vi "PWA_Setup_Panel.vi"(0 "Show Panel?":bool, 1 "Check Calib file?":bool, 2 "OK":T1, 3 "Incoming Setup String":string) -> (7 "Outgoing Setup String":string)   [LabVIEW 2013]
uses:
  Controls/ok_button.ctl
  File/Setup_Filetype.ctl
  Controls/Post_Process.ctl
  Controls/App_Global.ctl
  Controls/Inst_type.ctl
  Globals/Meas_global.vi
  PWAtasksGLOBAL.vi
panel:
  in  "Probe Rotated Thro' 180":bool
  in  "Software + buffering delay per pulse (s)":dbl=9.7e-06
  in  "Symbol":string
  in  "Pulse length \nx2 micro sec":i16=1 min=1 max=12
  in  "Clock Rate":bool
  in  "Gain":i16=1 min=1 max=12
  in  "Wire Current mA":i16(knob)=1 min=1 max=3 step=1 scale=1.0..3.0
  in  "Trigger -ve":dbl(knob)=1.0 min=0.0 max=5.0 scale=0.0..5.0 scale format="%#.2f"
  in  "Trigger +ve":dbl(knob)=1.0 min=0.0 max=5.0 scale=0.0..5.0 scale format="%#.2f"
  out "Calib Path from file":path
  in  "Use Latest":bool=TRUE
  in  "PWA Calib. File Path":path=path "/G5_1_HD/Users/paulhayden/Desktop/Labview test/PWA_Calib.xls"
  in  "Minimum TOF (mu.s)":i16=225
  in  "PWA Freq. (Hz)":dbl=30.0 min=0.0 max=50.0
  # "PELA Flow Instruments Ltd."
  # "TRIGGER LEVELS\n(volts)"
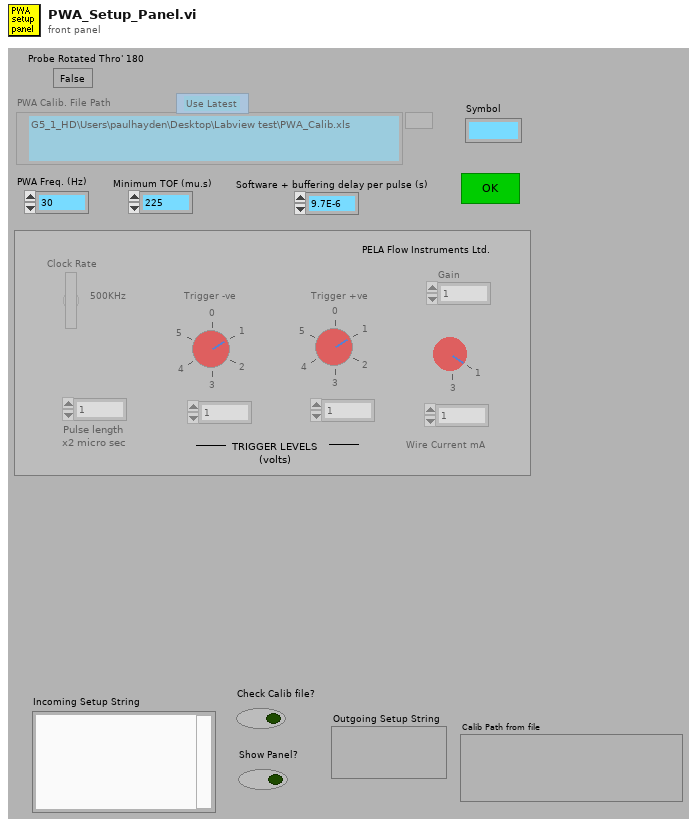
[diagram p1: front panel]
types:
  T1 = typedef "ok_button.ctl" = bool
  T2 = typedef "Setup_Filetype.ctl" = enum16{"Measurement Setups", "Calibration Setups", "General", "Results File Plotter Setups", "Speed Calib Tweaks"}
  T3 = typedef "Post_Process.ctl" = enum16{"Take New Data", "Post Process Raw Data File"}
  T4 = typedef "App_Global.ctl" = enum16{"Read Global", "Write to Global", "Initialise Array"}
  T5 = typedef "Inst_type.ctl" = enum16{"Propeller anemometer", "Raw voltage", "Pressure Transducer", "Pitot-static tube", "Preston tube", "Hot wire", "Cross wire 1", "Cross wire 2", "Generic Linear", "Generic Polynomial", "Generic BackPoly", "Fast FID", "Thermocouple", "Cold wire", "Pulsed Wire", "LDA Vel", "LDA Tran time", "LDA Arr time"}
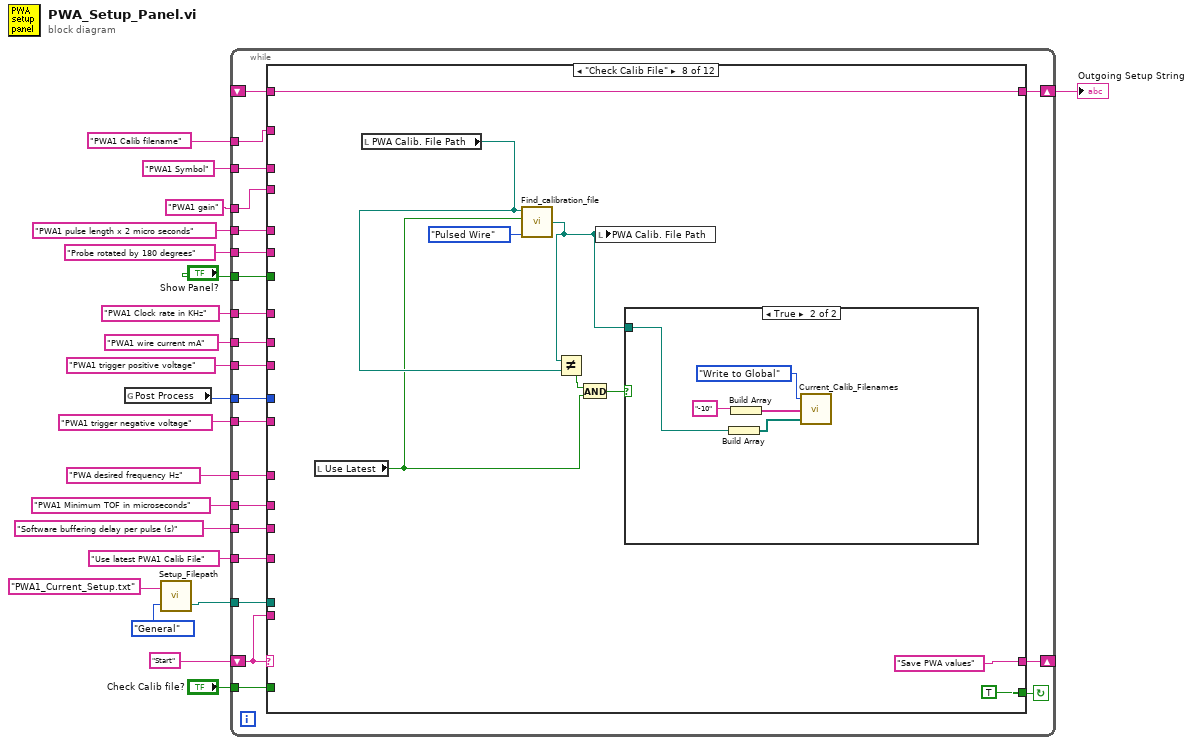
[diagram p0: block diagram]
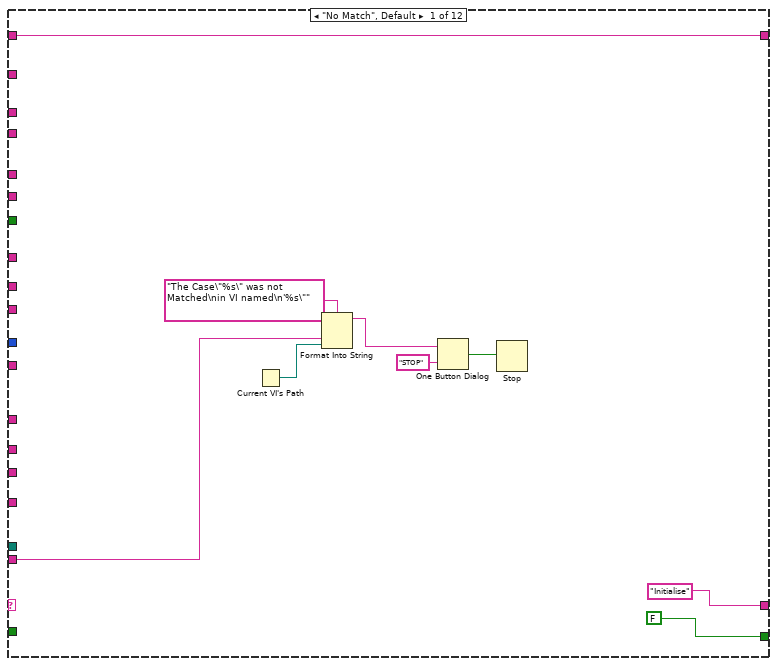
[diagram p2: hidden frame]
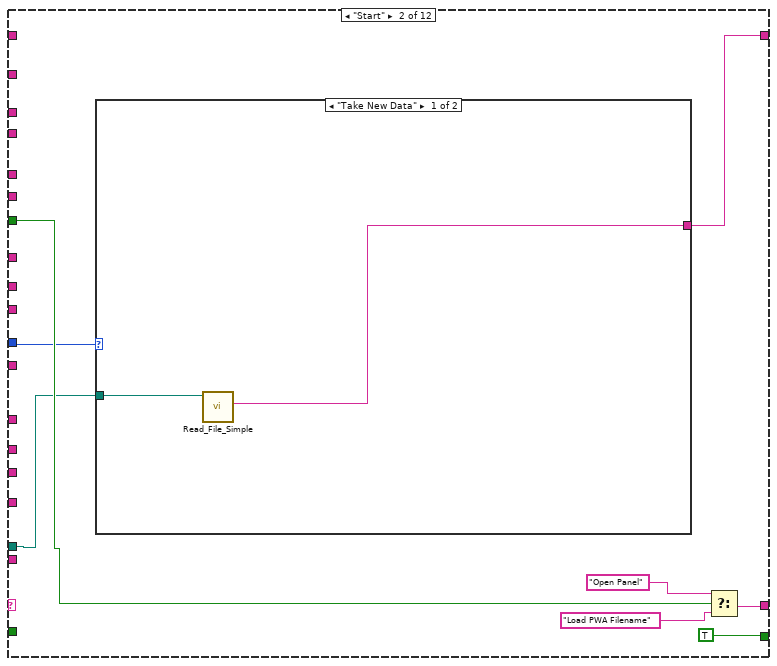
[diagram p3: hidden frame]
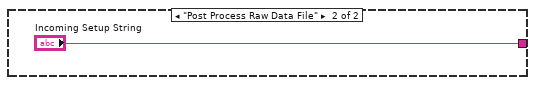
[diagram p4: hidden frame]
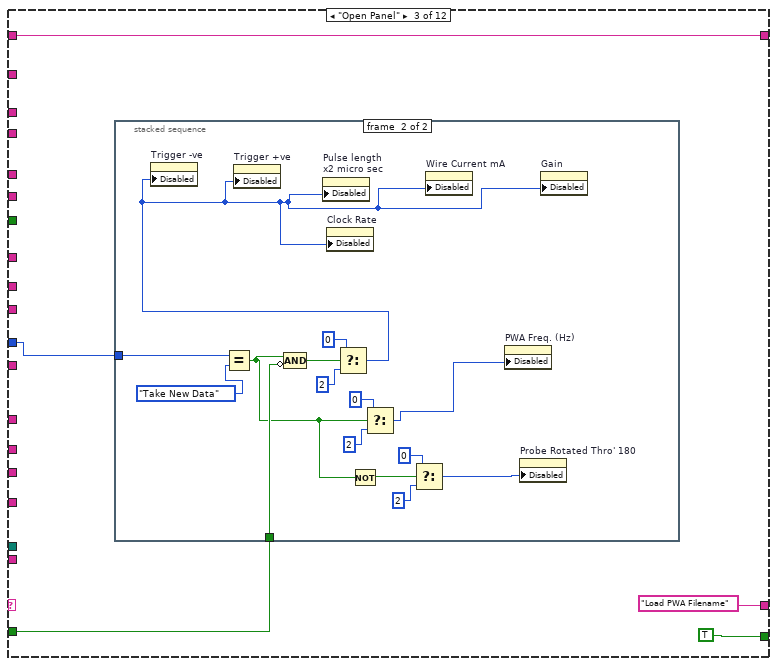
[diagram p5: hidden frame]
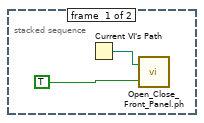
[diagram p6: hidden frame]
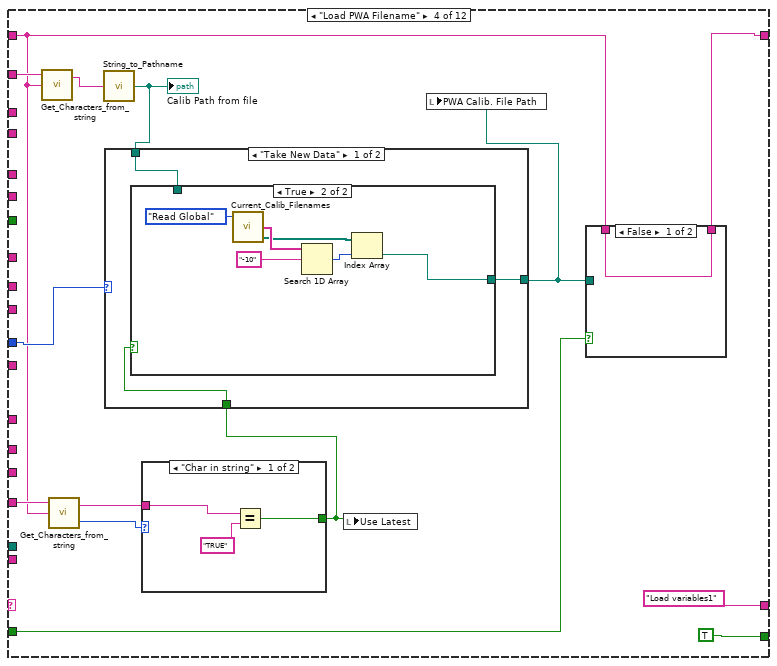
[diagram p7: hidden frame]
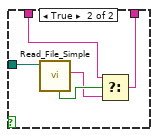
[diagram p8: hidden frame]
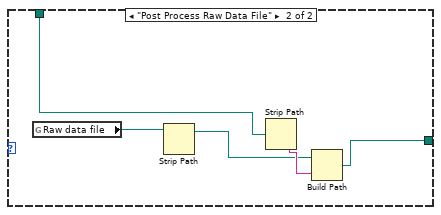
[diagram p10: hidden frame]
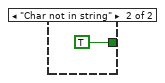
[diagram p11: hidden frame]
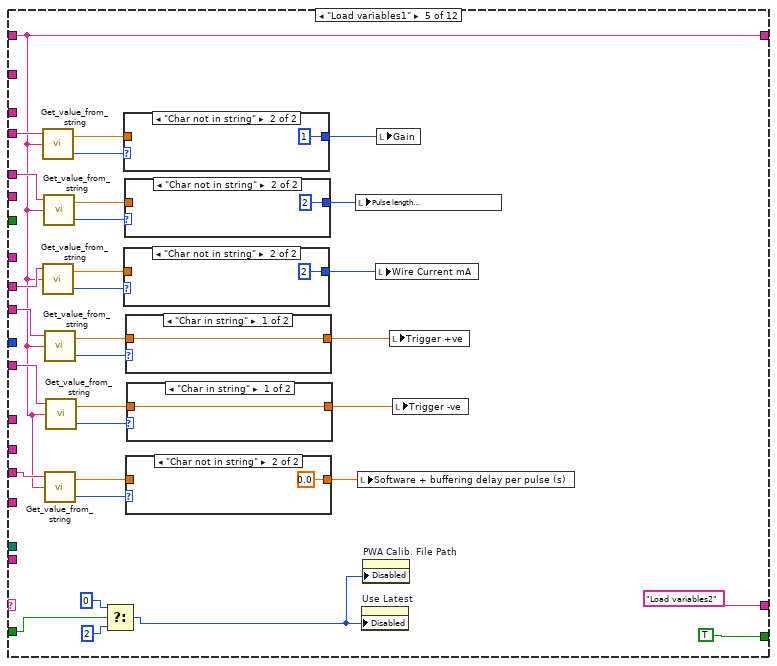
[diagram p12: hidden frame]
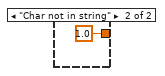
[diagram p14: hidden frame]
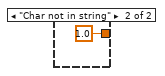
[diagram p15: hidden frame]
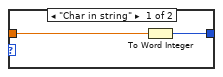
[diagram p16: hidden frame]
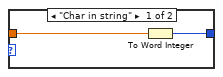
[diagram p17: hidden frame]
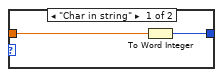
[diagram p18: hidden frame]
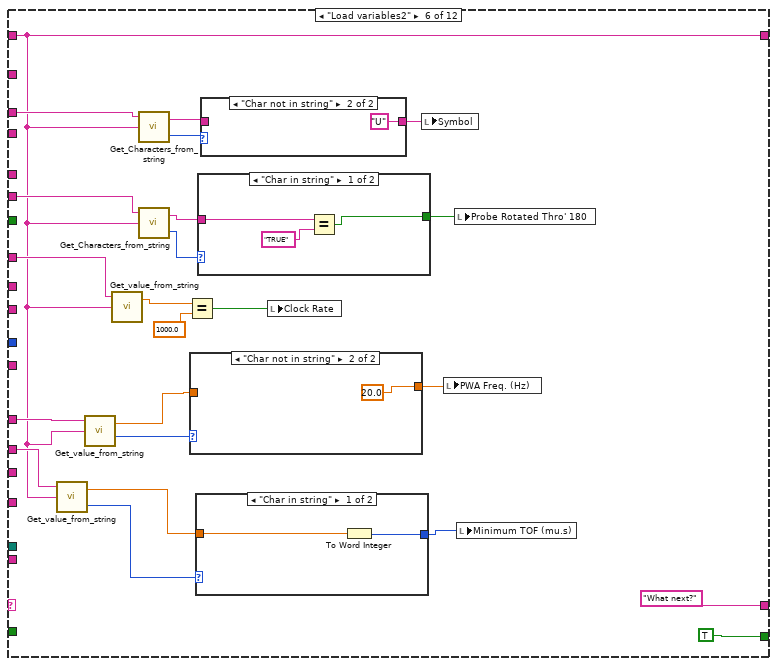
[diagram p19: hidden frame]
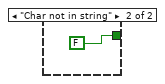
[diagram p20: hidden frame]
diagram:
  n1 = global read "Meas_global.vi" "Post Process"() -> (w19:T3)
  n2 = call "Setup_Filepath.vi"("Setup File Type"=Setup_Filetype."General", "Filename in"="PWA1_Current_Setup.txt" ("name or relative path")) -> ("Filename Out"=w1:path)  [unwired: 1 out]
  n3 = while {
    shift-left: "Start" -> [w41]
    shift-right: [w42] -> _
    tunnel: "Show Panel?" -> [w40]
    tunnel: w19 -> [w39]
    tunnel: "PWA1 Calib filename" -> [w37]
    tunnel: "Use latest PWA1 Calib File" -> [w38]
    tunnel: "PWA1 Minimum TOF in microseconds" -> [w36]
    tunnel: "PWA desired frequency Hz" -> [w35]
    tunnel: "Check Calib file?" -> [w34]
    tunnel: "PWA1 gain" -> [w33]
    tunnel: "PWA1 pulse length x 2 micro seconds" -> [w32]
    tunnel: "PWA1 wire current mA" -> [w31]
    tunnel: "PWA1 trigger positive voltage" -> [w30]
    tunnel: "PWA1 trigger negative voltage" -> [w29]
    tunnel: "PWA1 Clock rate in KHz" -> [w28]
    shift-right: [w27] -> w6
    shift-left: _ -> [w26]
    tunnel: "PWA1 Symbol" -> [w25]
    tunnel: w1 -> [w24]
    tunnel: "Software buffering delay per pulse (s)" -> [w23]
    tunnel: "Probe rotated by 180 degrees" -> [w22]
    stop <- w43 continue-if-true
    n4 = case shown="\"Check Calib File\"" w41 {
      tunnel: [FALSE TRUE TRUE TRUE TRUE TRUE TRUE TRUE ("Show Panel?") TRUE ("Show Panel?") TRUE ("Show Panel?") w331 FALSE ("Show Panel?")] -> w43
      tunnel: ["Initialise" w53 "Load PWA Filename" "Load variables1" "Load variables2" "What next?" w211 "Save PWA values" "2nd Save PWA values" "PWA Setup Summary" "Close Panel" "End"] -> w42
      tunnel: w41 -> [w47 _ _ _ _ _ _ _ _ _ _ _]
      tunnel: w40 -> [_ w59 _ _ _ _ _ _ _ _ w331 _]
      tunnel: w39 -> [_ w56 w66 w91 _ _ w213 _ _ _ _ w333]
      tunnel: w38 -> [_ _ _ w93 _ _ _ _ w269 _ _ _]
      tunnel: w37 -> [_ _ _ w96 _ _ _ _ w279 _ _ _]
      tunnel: w36 -> [_ _ _ _ _ w191 _ _ w277 _ _ _]
      tunnel: w35 -> [_ _ _ _ _ w190 _ _ w278 _ _ _]
      tunnel: w34 -> [_ _ w64 w88 w153 _ w209 _ _ _ _ _]
      tunnel: w33 -> [_ _ _ _ w146 _ _ _ _ w316 _ _]
      tunnel: w32 -> [_ _ _ _ w142 _ _ _ _ w300 _ _]
      tunnel: w31 -> [_ _ _ _ w130 _ _ _ _ w305 _ _]
      tunnel: w30 -> [_ _ _ _ w135 _ _ _ _ w302 _ _]
      tunnel: w29 -> [_ _ _ _ w131 _ _ _ _ w301 _ _]
      tunnel: w28 -> [_ _ _ _ _ w183 _ _ _ w311 _ _]
      tunnel: [w44 w55 w65 w86 w126 w174 w208 w241 w265 w291 w321 w337] -> w27
      tunnel: w26 -> [w44 _ w65 w87 w126 w174 w208 w241 _ w292 w321 w337]
      tunnel: w25 -> [_ _ _ _ _ w179 _ _ w263 _ _ _]
      tunnel: w24 -> [_ w54 _ _ _ _ _ _ _ _ _ w336]
      tunnel: w23 -> [_ _ _ _ w127 _ _ _ _ w289 _ _]
      tunnel: w22 -> [_ _ _ _ _ w175 _ _ w256 _ _ _]
      frame "No Match", Default {
        n5 = Current VI's Path() -> (path=w46:path)
        n6 = Format Into String(format string="The Case\"%s\" was not Matched\nin VI named\n'%s\"" ("Format String"), w47, w46) -> (resulting string=w50:string)  [unwired: 2 in, 1 out]
        n7 = One Button Dialog(message=w50, button name ("OK")="STOP") -> (true=w48:bool)
        n8 = Stop(stop? (T)=w48) -> ()
      }
      frame "Start" {
        n9 = case shown="\"Take New Data\"" w56 {
          tunnel: [w61 "Incoming Setup String"] -> w55
          tunnel: w54 -> [w62 _]
          frame "Take New Data" {
            n10 = call "Read_File_Simple.vi"("Filename"=w62) -> ("string"=w61:string)  [unwired: 2 in, 7 out]
          }
          frame "Post Process Raw Data File" {
          }
        }
        n11 = Select(t="Open Panel", s=w59, f="Load PWA Filename") -> (s? t:f=w53:string)
      }
      frame "Open Panel" {
        n12 = stacked-sequence {
          tunnel: w66 -> [_ w85]
          tunnel: w64 -> [_ w80]
          frame #0 {
            n13 = Current VI's Path() -> (path=w70:path)
            n14 = call "Open_Close_Front_Panel.ph.vi"("Front Panel Window:Open"=TRUE, "VI path"=w70) -> ()  [unwired: 2 out]
          }
          frame #1 {
            n15 = Equal?(x=w85, y=Post_Process."Take New Data" ("Post Process")) -> (x = y?=w73:bool)
            n16 = Compound Arithmetic op=AND(w73, invert w80) -> (w79:bool)
            n17 = Select(t=u8 0 ("Disabled"), s=w79, f=u8 2) -> (s? t:f=w81:u8)
            n18 = property on="Trigger -ve" class="Knob (strict)"("Disabled"=w81) -> ()  [unwired: 2 in, 2 out]
            n19 = property on="Trigger +ve" class="Knob (strict)"("Disabled"=w81) -> ()  [unwired: 2 in, 2 out]
            n20 = property on="Pulse length \nx2 micro sec" class="DigNum (strict)"("Disabled"=w81) -> ()  [unwired: 2 in, 2 out]
            n21 = property on="Clock Rate" class="Bool (strict)"("Disabled"=w81) -> ()  [unwired: 2 in, 2 out]
            n22 = Not(x=w73) -> (.not. x?=w72:bool)
            n23 = Select(t=u8 0 ("Disabled"), s=w73, f=u8 2) -> (s? t:f=w76:u8)
            n24 = Select(t=u8 0 ("Disabled"), s=w72, f=u8 2) -> (s? t:f=w71:u8)
            n25 = property on="Wire Current mA" class="Knob (strict)"("Disabled"=w81) -> ()  [unwired: 2 in, 2 out]
            n26 = property on="PWA Freq. (Hz)" class="DigNum (strict)"("Disabled"=w76) -> ()  [unwired: 2 in, 2 out]
            n27 = property on="Probe Rotated Thro' 180" class="Bool (strict)"("Disabled"=w71) -> ()  [unwired: 2 in, 2 out]
            n28 = property on="Gain" class="DigNum (strict)"("Disabled"=w81) -> ()  [unwired: 2 in, 2 out]
          }
        }
      }
      frame "Load PWA Filename" {
        n29 = call "Get_Characters_from_string.vi"("Input string"=w87, "Variable name"=w96) -> ("Value"=w97:string)  [unwired: 1 in, 1 out]
        n30 = call "Get_Characters_from_string.vi"("Input string"=w87, "Variable name"=w93) -> ("Status"=w94:enum16{"Char in string", "Char not in string"}, "Value"=w95:string)  [unwired: 1 in]
        n31 = call "String_to_Pathname.vi"("Input String"=w97) -> ("path"=w92:path)
        "Calib Path from file" <- w92
        n32 = case shown="\"Char in string\"" w94 {
          tunnel: w95 -> [w123 _]
          tunnel: [w121 TRUE] -> w90
          frame "Char in string" {
            n33 = Equal?(x=w123, y="TRUE") -> (x = y?=w121:bool)
          }
          frame "Char not in string" {
          }
        }
        n34 = case shown="\"Take New Data\"" w91 {
          tunnel: [w107 w116] -> w89
          tunnel: w92 -> [w106 w119]
          tunnel: w90 -> [w108 _]
          frame "Take New Data" {
            n35 = case shown="True" w108 {
              tunnel: [w109 w114] -> w107
              tunnel: w106 -> [w109 _]
              frame False {
              }
              frame True {
                n36 = call "Current_Calib_Filenames.vi"("Mode"=App_Global."Read Global") -> ("Calib Filename Out"=w112:path[], "Channel Numbers Out"=w113:string[])  [unwired: 3 in]
                n37 = Search 1D Array(1D array=w113, element="-10") -> (index of element=w115:i32)  [unwired: 1 out]
                n38 = Index Array(array=w112, index=w115) -> (element=w114:path)
              }
            }
          }
          frame "Post Process Raw Data File" {
            n39 = global read "Meas_global.vi" "Raw data file"() -> (w120:path)
            n40 = Strip Path(path=w120) -> (stripped path=w117:path)  [unwired: 1 out]
            n41 = Strip Path(path=w119) -> (name=w118:string)  [unwired: 1 out]
            n42 = Build Path(base path=w117, name or relative path=w118) -> (appended path=w116:path)
          }
        }
        n43 = local write "Use Latest"(w90) -> ()
        n44 = local write "PWA Calib. File Path"(w89) -> ()
        n45 = case shown="False" w88 {
          tunnel: w89 -> [_ w105]
          tunnel: w87 -> [w100 w102]
          tunnel: [w100 w101] -> w86
          frame False {
          }
          frame True {
            n46 = call "Read_File_Simple.vi"("Filename"=w105) -> ("Error?"=w104:bool, "string"=w103:string)  [unwired: 2 in, 6 out]
            n47 = Select(t=w102, s=w104, f=w103) -> (s? t:f=w101:string)
          }
        }
      }
      frame "Load variables1" {
        n48 = call "Get_value_from_string.vi"("Input string"=w126, "Variable name"=w146) -> ("Status"=w148:enum16{"Char in string", "Char not in string"}, "Value"=w149:dbl)  [unwired: 1 in]
        n49 = call "Get_value_from_string.vi"("Input string"=w126, "Variable name"=w130) -> ("Status"=w140:enum16{"Char in string", "Char not in string"}, "Value"=w141:dbl)  [unwired: 1 in]
        n50 = call "Get_value_from_string.vi"("Input string"=w126, "Variable name"=w142) -> ("Status"=w144:enum16{"Char in string", "Char not in string"}, "Value"=w143:dbl)  [unwired: 1 in]
        n51 = call "Get_value_from_string.vi"("Input string"=w126, "Variable name"=w135) -> ("Status"=w137:enum16{"Char in string", "Char not in string"}, "Value"=w136:dbl)  [unwired: 1 in]
        n52 = call "Get_value_from_string.vi"("Input string"=w126, "Variable name"=w127) -> ("Status"=w128:enum16{"Char in string", "Char not in string"}, "Value"=w125:dbl)  [unwired: 1 in]
        n53 = call "Get_value_from_string.vi"("Input string"=w126, "Variable name"=w131) -> ("Status"=w133:enum16{"Char in string", "Char not in string"}, "Value"=w134:dbl)  [unwired: 1 in]
        n54 = Select(t=u8 0 ("Disabled"), s=w153, f=u8 2 ("Disabled")) -> (s? t:f=w150:u8)
        n55 = case shown="\"Char not in string\"" w148 {
          tunnel: w149 -> [w169 _]
          tunnel: [w168 i16 1 ("PWA No. of Samples")] -> w147
          frame "Char in string" {
            n56 = To Word Integer(number=w169) -> (16bit integer=w168:i16)
          }
          frame "Char not in string" {
          }
        }
        n57 = case shown="\"Char not in string\"" w140 {
          tunnel: w141 -> [w163 _]
          tunnel: [w162 i16 2 ("PWA No. of Samples")] -> w139
          frame "Char in string" {
            n58 = To Word Integer(number=w163) -> (16bit integer=w162:i16)
          }
          frame "Char not in string" {
          }
        }
        n59 = case shown="\"Char not in string\"" w144 {
          tunnel: w143 -> [w166 _]
          tunnel: [w165 i16 2 ("PWA No. of Samples")] -> w145
          frame "Char in string" {
            n60 = To Word Integer(number=w166) -> (16bit integer=w165:i16)
          }
          frame "Char not in string" {
          }
        }
        n61 = case shown="\"Char in string\"" w137 {
          tunnel: w136 -> [w160 _]
          tunnel: [w160 1.0 ("Value")] -> w138
          frame "Char in string" {
          }
          frame "Char not in string" {
          }
        }
        n62 = case shown="\"Char not in string\"" w128 {
          tunnel: w125 -> [w156 _]
          tunnel: [w156 0.0 ("Value")] -> w129
          frame "Char in string" {
          }
          frame "Char not in string" {
          }
        }
        n63 = case shown="\"Char in string\"" w133 {
          tunnel: w134 -> [w158 _]
          tunnel: [w158 1.0 ("Value")] -> w132
          frame "Char in string" {
          }
          frame "Char not in string" {
          }
        }
        n64 = local write "Pulse length \nx2 micro sec"(w145) -> ()
        n65 = local write "Software + buffering delay per pulse (s)"(w129) -> ()
        n66 = property on="Use Latest" class="Bool (strict)"("Disabled"=w150) -> ()  [unwired: 2 in, 2 out]
        n67 = property on="PWA Calib. File Path" class="Path"("Disabled"=w150) -> ()  [unwired: 2 in, 2 out]
        n68 = local write "Wire Current mA"(w139) -> ()
        n69 = local write "Gain"(w147) -> ()
        n70 = local write "Trigger +ve"(w138) -> ()
        n71 = local write "Trigger -ve"(w132) -> ()
      }
      frame "Load variables2" {
        n72 = call "Get_value_from_string.vi"("Input string"=w174, "Variable name"=w191) -> ("Status"=w186:enum16{"Char in string", "Char not in string"}, "Value"=w185:dbl)  [unwired: 1 in]
        n73 = call "Get_value_from_string.vi"("Input string"=w174, "Variable name"=w190) -> ("Status"=w189:enum16{"Char in string", "Char not in string"}, "Value"=w188:dbl)  [unwired: 1 in]
        n74 = call "Get_value_from_string.vi"("Input string"=w174, "Variable name"=w183) -> ("Value"=w182:dbl)  [unwired: 1 in, 1 out]
        n75 = call "Get_Characters_from_string.vi"("Input string"=w174, "Variable name"=w179) -> ("Status"=w178:enum16{"Char in string", "Char not in string"}, "Value"=w177:string)  [unwired: 1 in]
        n76 = call "Get_Characters_from_string.vi"("Input string"=w174, "Variable name"=w175) -> ("Status"=w173:enum16{"Char in string", "Char not in string"}, "Value"=w171:string)  [unwired: 1 in]
        n77 = Equal?(x=w182, y=1000.0) -> (x = y?=w180:bool)
        n78 = case shown="\"Char not in string\"" w189 {
          tunnel: w188 -> [w203 _]
          tunnel: [w203 20.0 ("PWA No. of Samples")] -> w187
          frame "Char in string" {
          }
          frame "Char not in string" {
          }
        }
        n79 = case shown="\"Char in string\"" w186 {
          tunnel: w185 -> [w201 _]
          tunnel: [w200 i16 225 ("Minimum TOF (mu.s)")] -> w184
          frame "Char in string" {
            n80 = To Word Integer(number=w201) -> (16bit integer=w200:i16)
          }
          frame "Char not in string" {
          }
        }
        n81 = case shown="\"Char in string\"" w173 {
          tunnel: [w194 FALSE] -> w172
          tunnel: w171 -> [w196 _]
          frame "Char in string" {
            n82 = Equal?(x=w196, y="TRUE") -> (x = y?=w194:bool)
          }
          frame "Char not in string" {
          }
        }
        n83 = case shown="\"Char not in string\"" w178 {
          tunnel: w177 -> [w198 _]
          tunnel: [w198 "U" ("Value")] -> w176
          frame "Char in string" {
          }
          frame "Char not in string" {
          }
        }
        n84 = local write "Clock Rate"(w180) -> ()
        n85 = local write "Symbol"(w176) -> ()
        n86 = local write "PWA Freq. (Hz)"(w187) -> ()
        n87 = local write "Probe Rotated Thro' 180"(w172) -> ()
        n88 = local write "Minimum TOF (mu.s)"(w184) -> ()
      }
      frame "What next?" {
        n89 = local read "PWA Calib. File Path"() -> (w207:path)
        n90 = case shown="\"Take New Data\"" w213 {
          tunnel: [w223 w232] -> w205
          tunnel: w207 -> [w222 w235]
          tunnel: "Use Latest" -> [w224 _]
          frame "Take New Data" {
            n91 = case shown="True" w224 {
              tunnel: [w225 w230] -> w223
              tunnel: w222 -> [w225 _]
              frame False {
              }
              frame True {
                n92 = call "Current_Calib_Filenames.vi"("Mode"=App_Global."Read Global") -> ("Calib Filename Out"=w228:path[], "Channel Numbers Out"=w229:string[])  [unwired: 3 in]
                n93 = Search 1D Array(1D array=w229, element="-10") -> (index of element=w231:i32)  [unwired: 1 out]
                n94 = Index Array(array=w228, index=w231) -> (element=w230:path)
              }
            }
          }
          frame "Post Process Raw Data File" {
            n95 = global read "Meas_global.vi" "Raw data file"() -> (w236:path)
            n96 = Strip Path(path=w236) -> (stripped path=w233:path)  [unwired: 1 out]
            n97 = Strip Path(path=w235) -> (name=w234:string)  [unwired: 1 out]
            n98 = Build Path(base path=w233, name or relative path=w234) -> (appended path=w232:path)
          }
        }
        n99 = case shown="True" "OK" {
          tunnel: ["What next?" ("f") w219] -> w211
          tunnel: w209 -> [_ w218]
          frame False {
            n100 = Wait (ms)(milliseconds to wait=u32 300) -> ()  [unwired: 1 out]
          }
          frame True {
            n101 = Select(t="Check Calib File", s=w218, f="Save PWA values") -> (s? t:f=w219:string)
          }
        }
        n102 = Not Equal?(x=w207, y=w205) -> (x != y?=w206:bool)
        n103 = case shown="False" w206 {
          tunnel: w205 -> [_ w215]
          frame False {
          }
          frame True {
            n104 = local write "PWA Calib. File Path"(w215) -> ()
          }
        }
      }
      frame "Check Calib File" {
        n105 = local read "Use Latest"() -> (w237:bool)
        n106 = local read "PWA Calib. File Path"() -> (w240:path)
        n107 = call "Find_calibration_file.vi"("Inst type"=Inst_type."Pulsed Wire", "Use Latest Calib"=w237, "filename"=w240) -> ("filename out"=w239:path)  [unwired: 1 in]
        n108 = Not Equal?(x=w239, y=w240) -> (x != y?=w243:bool)
        n109 = And(x=w243, y=w237) -> (x .and. y?=w242:bool)
        n110 = local write "PWA Calib. File Path"(w239) -> ()
        n111 = case shown="True" w242 {
          tunnel: w239 -> [_ w250]
          frame False {
          }
          frame True {
            n112 = Build Array(w250) -> (w249:path[])
            n113 = Build Array("-10") -> (w248:string[])
            n114 = call "Current_Calib_Filenames.vi"("Calib Filename"=w249, "Channel Numbers"=w248, "Mode"=App_Global."Write to Global") -> ()  [unwired: 1 in, 2 out]
          }
        }
      }
      frame "Save PWA values" {
        n115 = local read "Use Latest"() -> (w273:bool)
        n116 = global write "PWAtasksGLOBAL.vi" "PWA Freq. (Hz)"("PWA Freq. (Hz)") -> ()
        n117 = global write "PWAtasksGLOBAL.vi" "PWA Calib. File Path"("PWA Calib. File Path") -> ()
        n118 = Select(t="TRUE", s=w273, f="FALSE") -> (s? t:f=w270:string)
        n119 = global write "PWAtasksGLOBAL.vi" "PWA Symbol"("Symbol") -> ()
        n120 = call "Characters_to_string.vi"("Characters to write"="Symbol", "Label for characters"=w263) -> ("Output string"=w262:string)
        n121 = call "Characters_to_string.vi"("Characters to write"=w270, "Label for characters"=w269) -> ("Output string"=w268:string)
        n122 = call "Value_to_string.vi"("Value"="PWA Freq. (Hz)", "Label for value"=w278) -> ("Output string"=w275:string)  [unwired: 1 in]
        n123 = global write "PWAtasksGLOBAL.vi" "Probe Rotated Thro' 180"("Probe Rotated Thro' 180") -> ()
        n124 = call "Path_2_String.vi"("Real Path"="PWA Calib. File Path") -> ("Path String"=w280:string)
        n125 = Select(t="TRUE" ("y"), s="Probe Rotated Thro' 180", f="FALSE") -> (s? t:f=w252:string)
        n126 = call "Characters_to_string.vi"("Characters to write"=w252, "Label for characters"=w256) -> ("Output string"=w253:string)
        n127 = call "Characters_to_string.vi"("Characters to write"=w280, "Label for characters"=w279) -> ("Output string"=w276:string)
        n128 = local read "Clock Rate"() -> (w260:bool)
        n129 = case shown="True" w260 {
          tunnel: [w283 w287] -> w259
          tunnel: [w282 w287] -> w258
          tunnel: "Minimum TOF (mu.s)" -> [w285 w287]
          frame False {
            w284 = i16 2 ("y")
            n130 = Divide(x=w285, y=w284) -> (x/y=w286:dbl)
            n131 = To Word Integer(number=w286) -> (16bit integer=w283:i16)
            n132 = Multiply(x=w283, y=w284) -> (x*y=w282:i16)
          }
          frame True {
          }
        }
        n133 = call "Value_to_string.vi"("Value"=w258, "Label for value"=w277) -> ("Output string"=w274:string)  [unwired: 1 in]
        n134 = Concatenate Strings(w276, w262, w253, w275, w274, w268) -> (w265:string)
        n135 = global write "PWAtasksGLOBAL.vi" "Minimum TOF Index"(w259) -> ()
      }
      frame "2nd Save PWA values" {
        n136 = Select(t=1000.0, s="Clock Rate", f=500.0) -> (s? t:f=w310:dbl)
        n137 = call "Value_to_string.vi"("Value"="Gain", "Label for value"=w316) -> ("Output string"=w298:string)  [unwired: 1 in]
        n138 = call "Value_to_string.vi"("Value"="Trigger -ve", "Label for value"=w301) -> ("Output string"=w293:string)  [unwired: 1 in]
        n139 = call "Value_to_string.vi"("Value"="Wire Current mA", "Label for value"=w305) -> ("Output string"=w295:string)  [unwired: 1 in]
        n140 = call "Value_to_string.vi"("Value"="Trigger +ve", "Label for value"=w302) -> ("Output string"=w294:string)  [unwired: 1 in]
        n141 = call "Value_to_string.vi"("Value"="Pulse length \nx2 micro sec", "Label for value"=w300) -> ("Output string"=w297:string)  [unwired: 1 in]
        n142 = call "Value_to_string.vi"("Value"=w310, "Label for value"=w311) -> ("Output string"=w296:string)  [unwired: 1 in]
        n143 = Multiply(x=w310, y=1000.0) -> (x*y=w308:dbl)
        n144 = Reciprocal(x=w308) -> (1/x=w307:dbl)
        n145 = call "Value_to_string.vi"("Value"="Software + buffering delay per pulse (s)", "Label for value"=w289) -> ("Output string"=w288:string)  [unwired: 1 in]
        n146 = global write "PWAtasksGLOBAL.vi" "PWA Seconds per clock pulse"(w307) -> ()
        n147 = Concatenate Strings(w292, w298, w297, w296, w295, w294, w293, w288) -> (w291:string)
      }
      frame "PWA Setup Summary" {
        n148 = local read "Pulse length \nx2 micro sec"() -> (w326:i16)
        n149 = local read "Wire Current mA"() -> (w325:i16)
        n150 = local read "Clock Rate"() -> (w330:bool)
        n151 = local read "Trigger -ve"() -> (w328:dbl)
        n152 = local read "Trigger +ve"() -> (w327:dbl)
        n153 = local read "Gain"() -> (w324:i16)
        n154 = Select(t="1MHz", s=w330, f="500KHz") -> (s? t:f=w329:string)
        n155 = Format Into String(format string="Clock=%s; Trig -ve=%.2f; Trig +ve=%.2f; Pulse length=%dx2micro sec; wire current=%dmA; Gain=%d", w329, w328, w327, w326, w325, w324) -> (resulting string=w322:string)  [unwired: 2 in, 1 out]
        n156 = global write "PWAtasksGLOBAL.vi" "PWA Setup summary"(w322) -> ()
      }
      frame "Close Panel" {
        n157 = case shown="\"Take New Data\"" w333 {
          tunnel: w337 -> [w342 _]
          tunnel: w336 -> [w341 _]
          frame "Take New Data" {
            w340 = FALSE  # append to file? (new file:F)
            n158 = call "Write_File_Simple.vi"("append to file? (new file:F)"=w340, "character string"=w342, "file path"=w341) -> ()  [unwired: 2 out]
          }
          frame "Post Process Raw Data File" {
          }
        }
        n159 = Current VI's Path() -> (path=w335:path)
        n160 = call "Open_Close_Front_Panel.ph.vi"("Front Panel Window:Open"=FALSE, "VI path"=w335) -> ()  [unwired: 2 out]
      }
    }
  }
  "Outgoing Setup String" <- w6
